vi "ListFiles.vi"(8 "error in (no error)":errorcluster, 11 "Google Drive Service Ref In":refnum<k24>) -> (0 "error out":errorcluster, 2 "Files":refnum<k24>[](array[refnum]))   [LabVIEW 2016, in "GDrive.lvlib"]
doc: "This VI will output an array of file references, generated from the contents of the User's Google Drive"
uses:
  GDrive.lvlib
  C:/Users/motoole/Desktop/VC OToolekit/Dependencies/Google.Apis.Drive.v3.dll
  Dependencies/Google.Apis.Drive.v3.dll
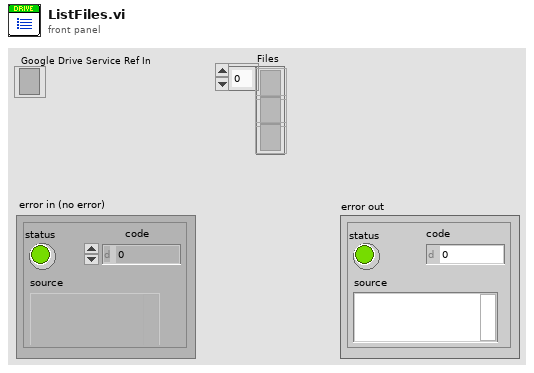
[diagram p1: front panel]
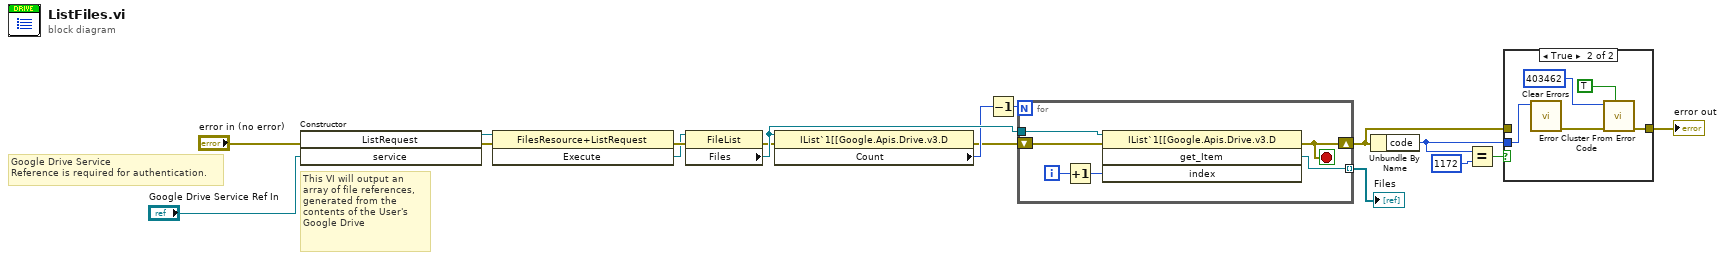
[diagram p0: block diagram]
diagram:
  # "Google Drive Service \nReference is required for authentication."
  # "This VI will output an array of file references, generated from the contents of the User's Google Drive"
  n1 = constructor class="FilesResource+ListRequest"(error in="error in (no error)", "service"="Google Drive Service Ref In") -> (reference out=w12:refnum<k24>, error out=w13:errorcluster)  [unwired: 2 in, 2 out]
  n2 = invoke class="FilesResource+ListRequest" method="Execute"(reference=w12, error in=w13) -> (error out=w14:errorcluster, "Execute"=w11:refnum<k24>)  [unwired: 1 in, 1 out]
  n3 = property class="FileList"(reference=w11, error in=w14) -> (error out=w15:errorcluster, "Files"=w17:refnum<k24>)  [unwired: 1 out]
  n4 = property class="IList`1[[Google.Apis.Drive.v3.D"(reference=w17, error in=w15) -> (error out=w1:errorcluster, "Count"=w2:i32)  [unwired: 1 out]
  n5 = Decrement(x=w2) -> (x-1=w3:i32)
  n6 = for {
    N: w3 -> [_]
    tunnel: w17 -> [w21]
    tunnel: [w20] -> w9 mode=indexing
    shift-right: [w19] -> w6
    shift-left: w1 -> [w18]
    i -> [w23]
    stop <- w19 stop-if-true
    n7 = Increment(x=w23) -> (x+1=w22:i32)
    n8 = invoke class="IList`1[[Google.Apis.Drive.v3.D" method="get_Item"(reference=w21, error in=w18, "index"=w22) -> (error out=w19:errorcluster, "get_Item"=w20:refnum<k24>)  [unwired: 1 in, 2 out]
  }
  "Files" <- w9
  n9 = Unbundle By Name(w6) -> ("code"=w4:i32)
  n10 = Equal?(x=w4, y=1172) -> (x = y?=w7:bool)
  n11 = case shown="True" w7 {
    tunnel: [w24 w27] -> w5
    tunnel: w6 -> [w24 _]
    tunnel: w4 -> [_ w29]
    frame False {
    }
    frame True {
      n12 = call <vilib>:"Clear Errors.vi"("specific error code to clear (0: all)"=w29) -> ("error out"=w28:errorcluster)  [unwired: 5 in, 1 out]
      n13 = call <vilib>:"Error Cluster From Error Code.vi"("show call chain? (False)"=TRUE, "error in (no error)"=w28, "error code (0)"=403462) -> ("error out"=w27:errorcluster)  [unwired: 6 in]
    }
  }
  "error out" <- w5
